vi "Configure Device.vi"(8 "error in (no error)":errorcluster, 10 "Max beams":dbl, 11 "WS5100 in":refnum<class "WS5100.lvclass">) -> (0 "error out":errorcluster, 3 "WS5100 out":refnum<class "WS5100.lvclass">)   [LabVIEW 2020, in "WS5100.lvclass"]
uses:
  WS5100.lvclass
  C:/Sandbox/Git_Sandbox/WiSpry Test Framework source code (LV20)/WiSpry Test Framework/Devices/NI DAQmx/NI DAQmx.lvclass
panel:
  in  "In use?":bool[](array[boolean])=[TRUE, TRUE, TRUE]
  in  "RFx 2":bool[](array[boolean])=[TRUE, TRUE, TRUE, TRUE]
  in  "RFx":bool[](array[boolean])=[TRUE, TRUE, TRUE, TRUE]
  in  "DAQmx line names":T1(array[cluster])=[{"lines"="Dev2/port0/line0", "Function"="Vdd", "Function"=enum."Vdd"}, {"lines"="Dev2/port1/line5", "Function"="Ctrl1", "Function"=enum."Control 1"}, {"lines"="Dev2/port2/line4", "Function"="Ctrl2", "Function"=enum."Control 2"}]
  in  "OK Button":bool
  # "RF1\nRF2\nRF3\nRF4"
  # "RFc"
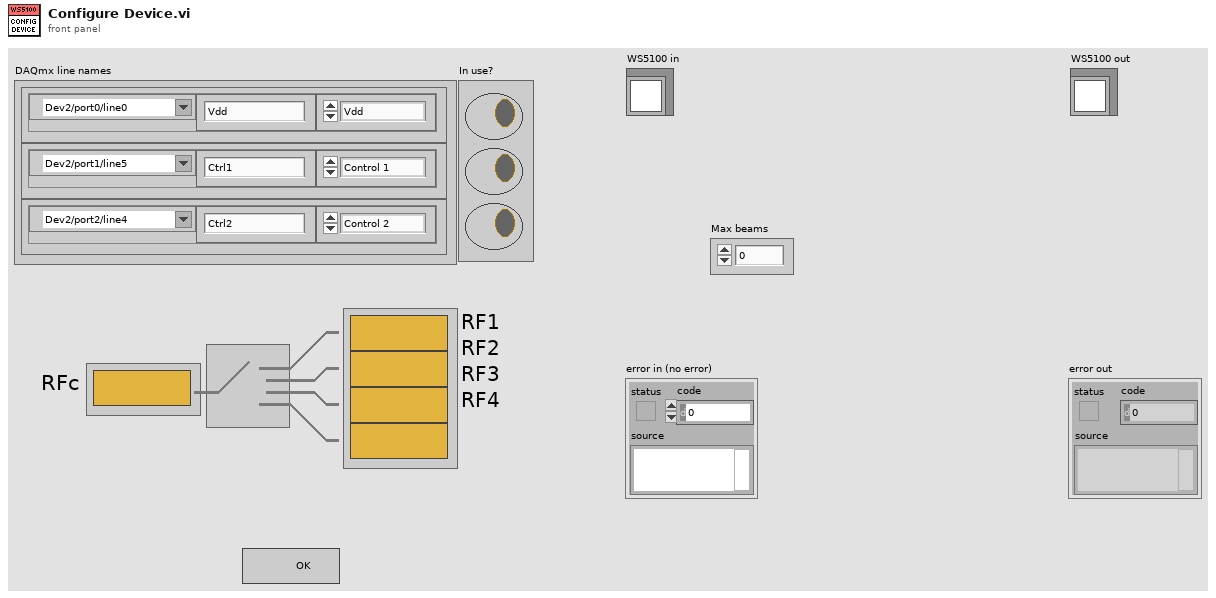
[diagram p1: front panel]
types:
  T1 = cluster{"lines":tag, "Function":string, "Function":enum16{"Vdd", "Control 0", "Control 1", "Control 2", "Control 3"}}[]
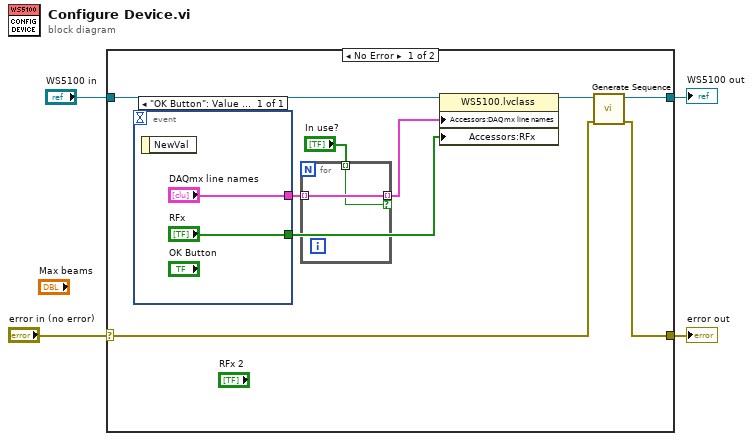
[diagram p0: block diagram]
diagram:
  n1 = case shown="No Error" "error in (no error)" {
    selector: "error in (no error)" -> [w9 w19]
    tunnel: [w8 w19] -> w3
    tunnel: [w10 w18] -> w2
    tunnel: "WS5100 in" -> [w13 w18]
    frame No Error {
      n2 = event shown="[0] \"OK Button\": Value Change" {
        selector: _ -> [_]
        dyn-events: _ -> [_]
        timeout: _ -> [_]
        tunnel: ["DAQmx line names"] -> w7
        tunnel: ["RFx"] -> w12
        event "OK Button": Value Change {
          n3 = event-data() -> ()  [unwired: 1 in, 1 out]
        }
      }
      n4 = for {
        tunnel: w7 -> [w15] mode=indexing
        tunnel: "In use?" -> [w14] mode=indexing
        tunnel: [w15] -> w5 mode=indexing if=w14
      }
      n5 = property class="WS5100.lvclass"(reference=w13, "Accessors:DAQmx line names"=w5, "Accessors:RFx"=w12) -> (reference out=w11:refnum<class "WS5100.lvclass">)  [unwired: 1 in, 1 out]
      n6 = call-dynamic "Generate Sequence.vi"("error in (no error)"=w9, "WS5100 in"=w11) -> ("error out"=w8:errorcluster, "WS5100 out"=w10:refnum<class "WS5100.lvclass">)  [unwired: 8 in]
    }
    frame Error {
    }
  }
  "error out" <- w3
  "WS5100 out" <- w2
